vi "test Get Base 10.vi"(11 "Test Case In":refnum<class "test Electronic Datasheet.lvclass">) -> (0 "error out":errorcluster, 3 "Test Case Out":refnum<class "test Electronic Datasheet.lvclass">)   [LabVIEW 2024, in "Test Utilities.lvclass"]
uses:
  Test Utilities.lvclass
  Test Utilities.lvclass/Test Utilities.ctl
  EDS-File-Viewer/Tests/source/test Electronic Datasheet/test Electronic Datasheet.lvclass
  <vilib>/Astemes/LUnit/Test Case.lvclass
  source/CANopen.lvlib
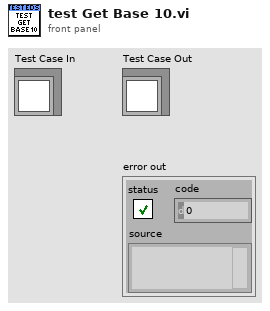
[diagram p1: front panel]
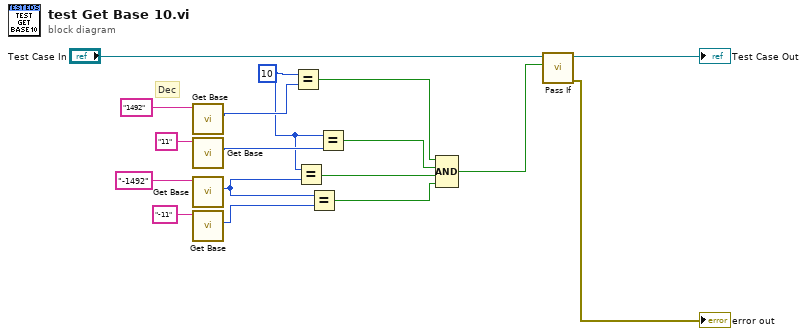
[diagram p0: block diagram]
diagram:
  w6 = u8 10
  # "Dec"
  n1 = call "Get Base.vi"("Default Value"="1492") -> ("Number Base"=w12:u8)  [unwired: 8 in, 2 out]
  n2 = call "Get Base.vi"("Default Value"="11") -> ("Number Base"=w11:u8)  [unwired: 8 in, 2 out]
  n3 = call "Get Base.vi"("Default Value"="-1492") -> ("Number Base"=w7:u8)  [unwired: 8 in, 2 out]
  n4 = call "Get Base.vi"("Default Value"="-11") -> ("Number Base"=w8:u8)  [unwired: 8 in, 2 out]
  n5 = Equal?(x=w6, y=w12) -> (x = y?=w5:bool)
  n6 = Equal?(x=w6, y=w7) -> (x = y?=w3:bool)
  n7 = Equal?(x=w7, y=w8) -> (x = y?=w2:bool)
  n8 = Equal?(x=w6, y=w11) -> (x = y?=w4:bool)
  n9 = Compound Arithmetic op=AND(w5, w4, w3, w2) -> (w1:bool)
  n10 = call <vilib>:"Pass If.vi"("Pass?"=w1, "LUnit Test Case In"="Test Case In") -> ("error out"=→"error out":errorcluster, "LUnit Test Case Out"=→"Test Case Out":refnum<class "test Electronic Datasheet.lvclass">)  [unwired: 8 in]
